vi "setChamber.vi"(8 "error in (no error)":errorcluster, 10 "Action":string, 11 "Instrument.Cryostat in":refnum<class "Instrument.Cryostat.lvclass">) -> (0 "error out":errorcluster, 3 "Instrument.Cryostat out":refnum<class "Instrument.Cryostat.lvclass">)   [LabVIEW 2019, in "Instrument.Cryostat.lvclass"]
uses:
  Instrument.Cryostat.lvclass
  Instrument/Instrument.lvclass
  9a542a78-1792-4c73-ab34-a6bd87c280a1.vi
  C:/Users/patrick/Documents/GitHub/Instrument-Framework/lvsrc/Instrument/Instrument.lvclass
  C:/Program Files (x86)/National Instruments/LabVIEW 2019/vi.lib/JKI/JKI SMO/SMO/SMO.lvclass
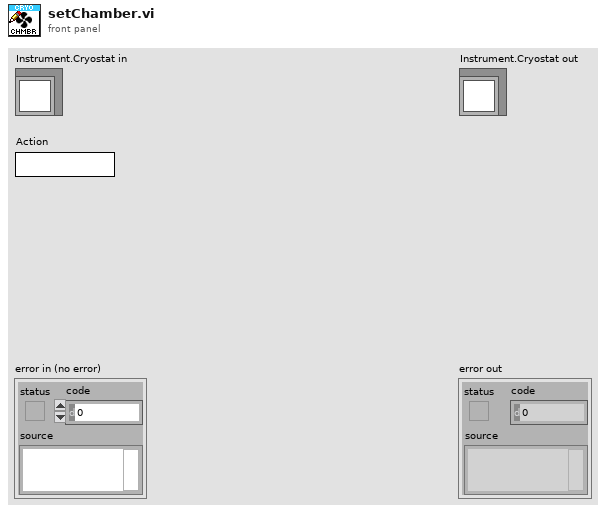
[diagram p1: front panel]
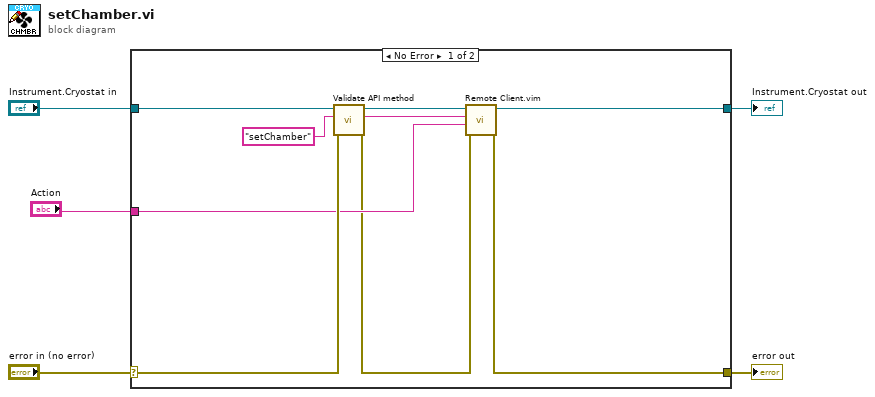
[diagram p0: block diagram]
diagram:
  n1 = case shown="No Error" "error in (no error)" {
    selector: "error in (no error)" -> [w9 w16]
    tunnel: [w8 w16] -> w4
    tunnel: [w10 w15] -> w2
    tunnel: "Instrument.Cryostat in" -> [w11 w15]
    tunnel: "Action" -> [w7 _]
    frame No Error {
      n2 = call "Validate API method.vi"("error in (no error)"=w9, "command in"="setChamber" ("error message (\"\")"), "Instrument in"=w11) -> ("error out"=w6:errorcluster, "command out"=w13:string, "Instrument out"=w12:refnum<class "Instrument.Cryostat.lvclass">)  [unwired: 6 in]
      n3 = call "Remote Client.vim"("error in (no error)"=w6, "params"=w7, "method"=w13, "Instrument in"=w12) -> ("error out"=w8:errorcluster, "Instrument out"=w10:refnum<class "Instrument.Cryostat.lvclass">)  [unwired: 4 in, 2 out]
    }
    frame Error {
    }
  }
  "error out" <- w4
  "Instrument.Cryostat out" <- w2
